vi "ADAM_scan_diagnostic.vi"() -> ()   [LabVIEW 2021]
uses:
  ADAM Client/Sub VIs/ADAM Controls/Ch_description_ADAM.ctl
  ADAM Client/Sub VIs/ADAM Controls/Module_type_ADAM.ctl
  ADAM Client/Sub VIs/ADAM Controls/Function_ADAM.ctl
  ADAM Client/Sub VIs/ADAM Controls/Channel_State.ctl
  ADAM Client/Sub VIs/ADAM Controls/Calib_type_ADAM.ctl
  ADAM Client/Sub VIs/ADAM Controls/Address.ctl
  ADAM_Global.vi
  Sub VI's/Channel_Description_Global.vi
panel:
  in  "deleteChannel":bool
  in  "reloadDescription":bool
  out "chTime(s)":dbl caption="Time taken" format="%_3ps"
  in  "Save Changes":bool
  in  "Simulate":enum32{"Scan Table", "Simulate"}(radio)
  in  "stop":bool
  in  "Value to Output":dbl format="%.2f"
  out "Value Read":dbl format="%.2f"
  out "Scan comment":string
  in  "Execute channel":bool
  in  "Select channel":bool
  in  "Ch Description":T1 {"Duty" format="%016b"; "D" format="%#_5g"; "C" format="%#_5g"; "B" format="%#_5g"; "A" format="%#_5g"}
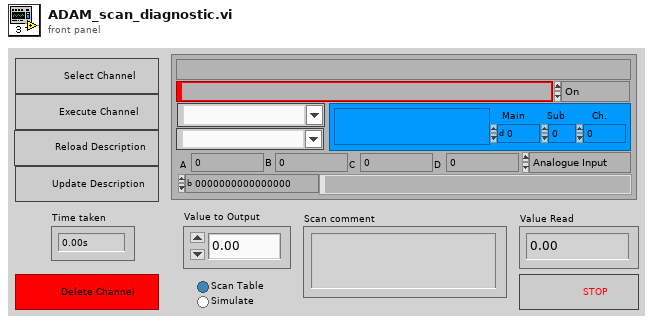
[diagram p1: front panel]
types:
  T1 = typedef "Ch_description_ADAM.ctl" = cluster{"Ch Name":string, "Type":T2, "Function":T3, "Ch State":T4, "Calibration type":T5, "A":dbl, "B":dbl, "C":dbl, "D":dbl, "Comments":string, "Address":T6, "String":string, "Duty":u16}
  T2 = typedef "Module_type_ADAM.ctl" = string
  T3 = typedef "Function_ADAM.ctl" = enum16{"Analogue Input", "Digital Input", "Event counter", "Event rate", "Analogue Output", "Digital Output", "Relay Output"}
  T4 = typedef "Channel_State.ctl" = enum16{"On", "Off", "Always On", "Always Off"}
  T5 = typedef "Calib_type_ADAM.ctl" = string
  T6 = typedef "Address.ctl" = cluster{"Main":i32, "Ch.":i32, "Sub":i32, "Port Name":string}
  T7 = enum16{"Load ADAM setup from excel file", "Save ADAM setup to excel file"}
  T8 = enum16{"Zero or one", "One", "Zero or more", "One or more"}
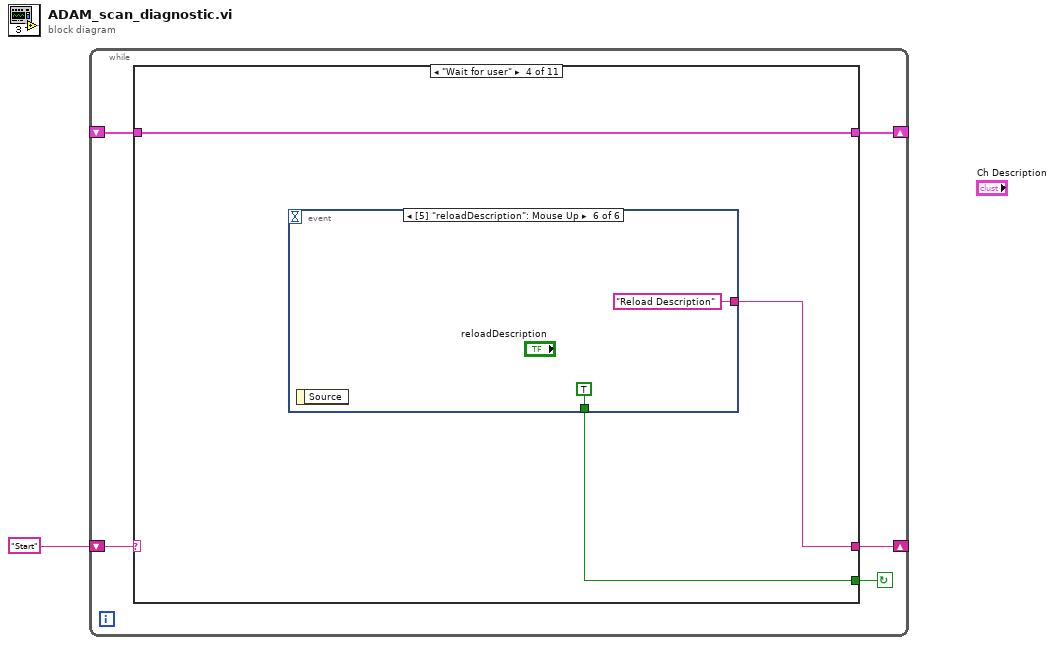
[diagram p0: block diagram]
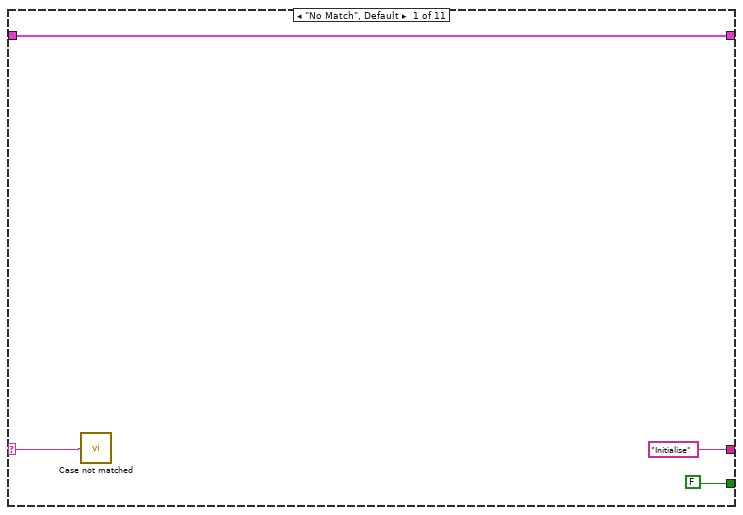
[diagram p2: hidden frame]
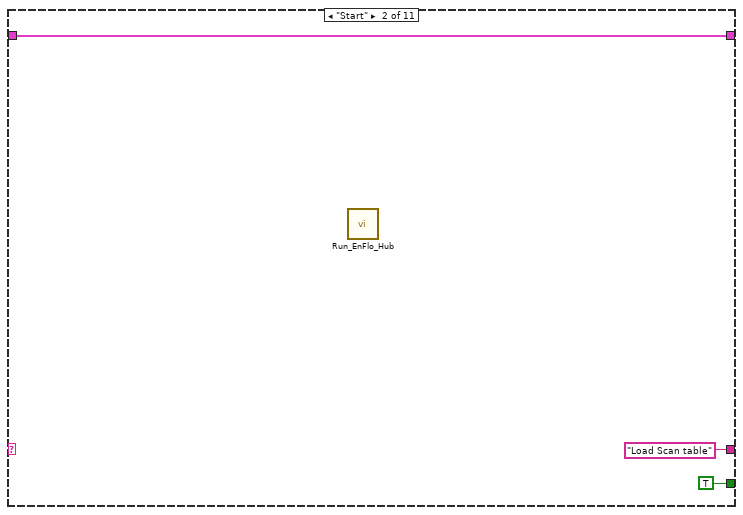
[diagram p3: hidden frame]
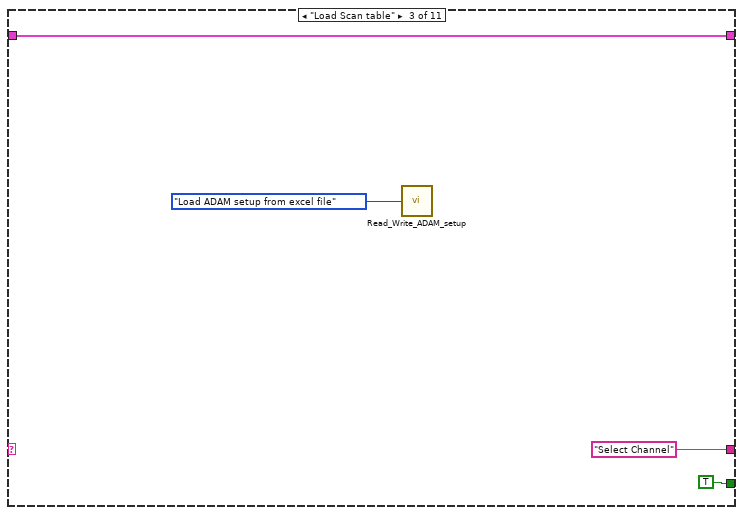
[diagram p4: hidden frame]
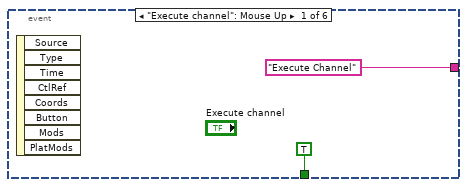
[diagram p5: hidden frame]
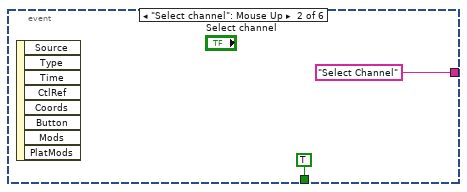
[diagram p6: hidden frame]
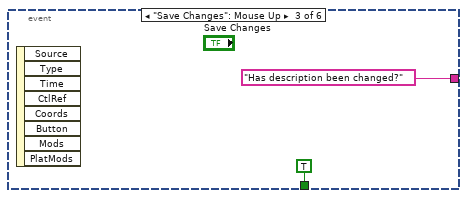
[diagram p7: hidden frame]
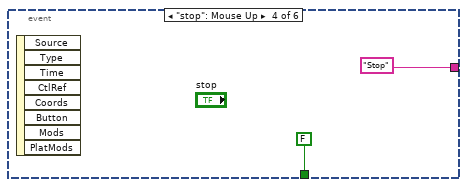
[diagram p8: hidden frame]
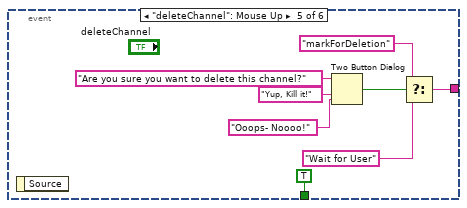
[diagram p9: hidden frame]
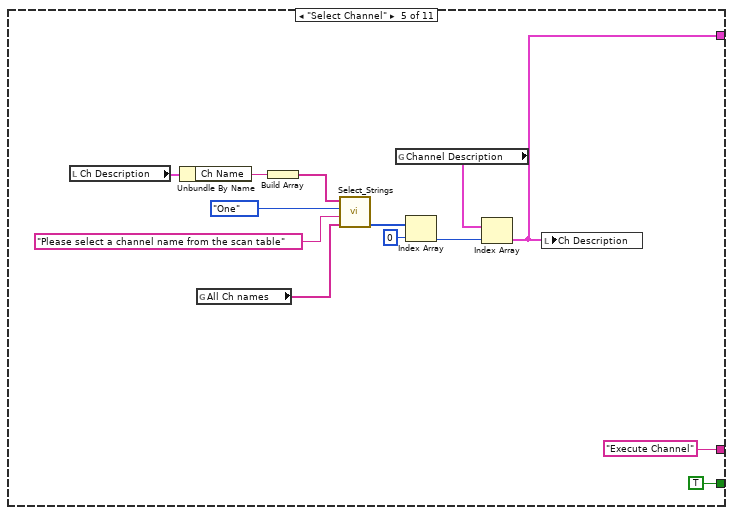
[diagram p10: hidden frame]
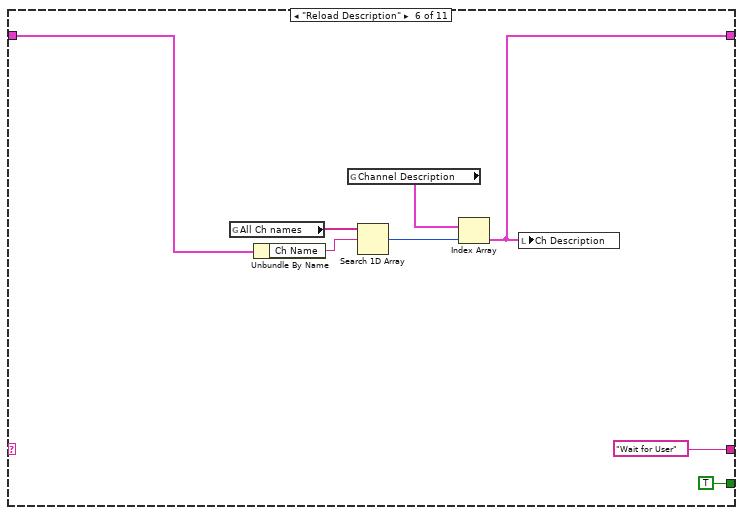
[diagram p11: hidden frame]
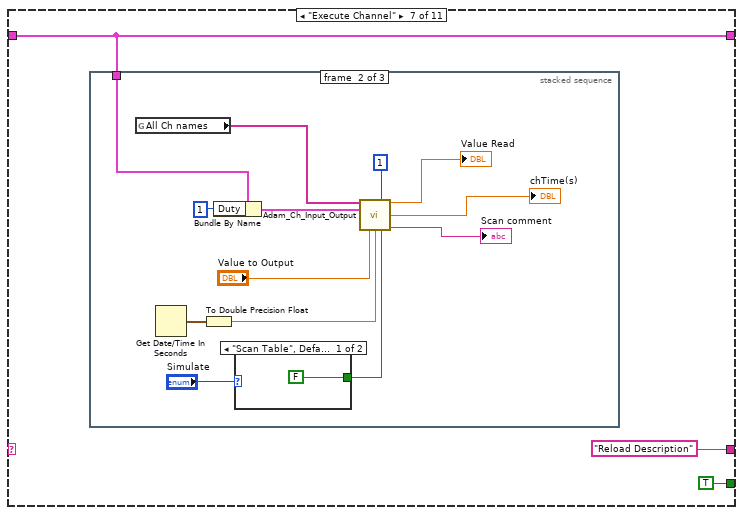
[diagram p12: hidden frame]
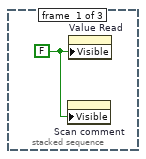
[diagram p13: hidden frame]
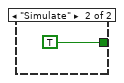
[diagram p14: hidden frame]
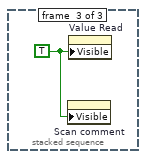
[diagram p15: hidden frame]
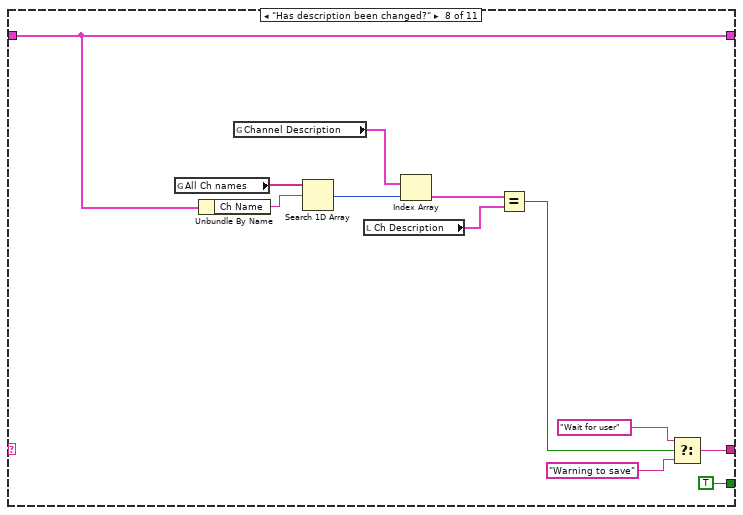
[diagram p16: hidden frame]
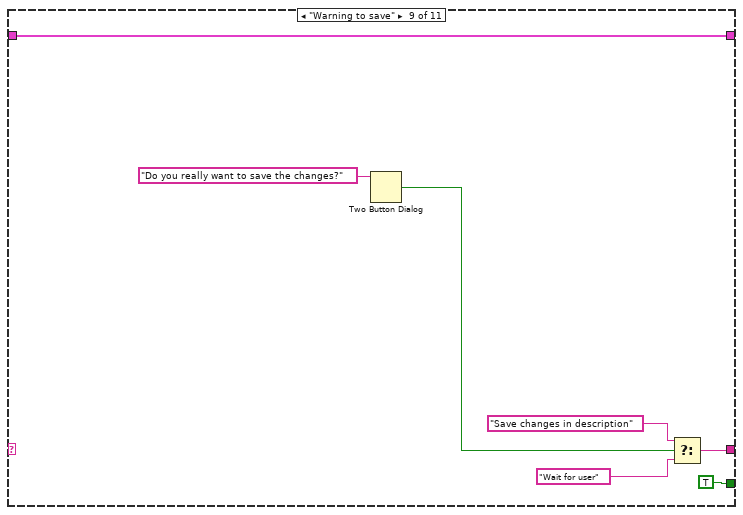
[diagram p17: hidden frame]
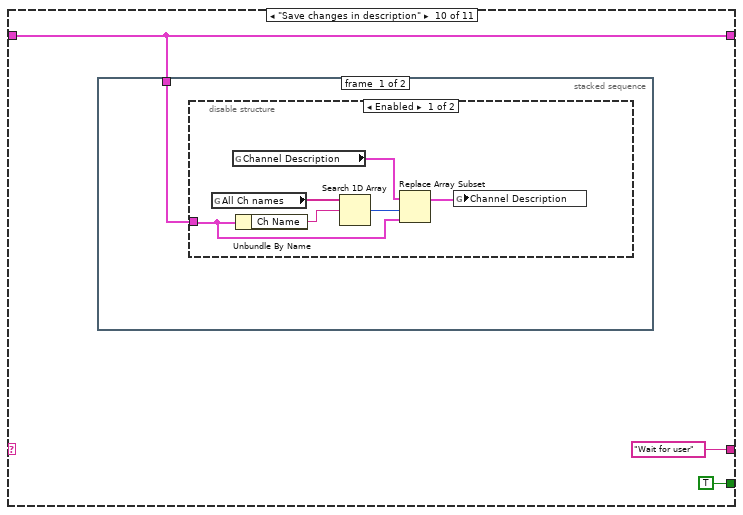
[diagram p18: hidden frame]
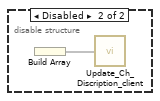
[diagram p19: hidden frame]
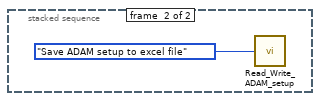
[diagram p20: hidden frame]
diagram:
  n1 = while {
    shift-left: "Start" -> [w4]
    shift-right: [w5] -> _
    shift-right: [w3] -> _
    shift-left: _ -> [w2]
    stop <- w6 continue-if-true
    n2 = case shown="\"Wait for user\"" w4 {
      selector: w4 -> [w8 _ _ _ _ _ _ _ _ _ _]
      tunnel: [FALSE TRUE TRUE w19 TRUE TRUE TRUE TRUE TRUE TRUE TRUE] -> w6
      tunnel: ["Initialise" "Load Scan table" "Select Channel" w20 "Execute Channel" "Wait for User" "Reload Description" w85 w97 "Wait for user" "Load Scan table"] -> w5
      tunnel: [w7 w11 w14 w18 w39 w52 w60 w81 w92 w99 w111] -> w3
      tunnel: w2 -> [w7 w11 w14 w18 _ w53 w60 w81 w92 w99 w111]
      frame "No Match", Default {
        n3 = call "Case not matched.vi"("Case Name not Matched"=w8) -> ()
      }
      frame "Start" {
        n4 = call "Run_EnFlo_Hub.vi"() -> ()  [unwired: 7 in, 1 out]
      }
      frame "Load Scan table" {
        n5 = call "Read_Write_ADAM_setup.vi"("Mode"=T7."Load ADAM setup from excel file") -> ()  [unwired: 4 in]
      }
      frame "Wait for user" {
        n6 = event shown="[5] \"reloadDescription\": Mouse Up" {
          selector: _ -> [_ _ _ _ _ _]
          dyn-events: _ -> [_ _ _ _ _ _]
          timeout: _ -> [_ _ _ _ _ _]
          tunnel: ["Execute Channel" "Select Channel" "Has description been changed?" "Stop" w33 "Reload Description"] -> w20
          tunnel: [TRUE TRUE TRUE FALSE TRUE TRUE] -> w19
          event "Execute channel": Mouse Up {
            n7 = event-data() -> ()  [unwired: 1 in, 8 out]
          }
          event "Select channel": Mouse Up {
            n8 = event-data() -> ()  [unwired: 1 in, 8 out]
          }
          event "Save Changes": Mouse Up {
            n9 = event-data() -> ()  [unwired: 1 in, 8 out]
          }
          event "stop": Mouse Up {
            n10 = event-data() -> ()  [unwired: 1 in, 8 out]
          }
          event "deleteChannel": Mouse Up {
            n11 = event-data() -> ()  [unwired: 1 in, 1 out]
            n12 = Two Button Dialog(message="Are you sure you want to delete this channel?", 1:"Ooops- Noooo!" ("F button name (\"Cancel\")"), 2:"Yup, Kill it!" ("T button name (\"OK\")")) -> (T button?=w32:bool)
            n13 = Select(t="markForDeletion", s=w32, f="Wait for User") -> (s? t:f=w33:string)
          }
          event "reloadDescription": Mouse Up {
            n14 = event-data() -> ()  [unwired: 1 in, 1 out]
          }
        }
      }
      frame "Select Channel" {
        n15 = local read "Ch Description"() -> (w43:T1)
        n16 = Unbundle By Name(w43) -> ("Ch Name"=w42:string)
        n17 = global read "ADAM_Global.vi" "All Ch names"() -> (w49:string[])
        n18 = Build Array(w42) -> (w41:string[])
        n19 = call "Select_Strings.vi"("Available Ch names"=w49, "Message"="Please select a channel name from the scan table", "Selector mode"=T8."One", "Desired Ch names (in)"=w41) -> ("Ch Indicies Chosen"=w45:i32[])  [unwired: 2 in, 2 out]
        n20 = global read "Channel_Description_Global.vi" "Channel Description"() -> (w44:T1[])
        n21 = Index Array(array=w45, index=0) -> (element=w40:i32)
        n22 = Index Array(array=w44, index=w40) -> (element=w39:T1)
        n23 = local write "Ch Description"(w39) -> ()
      }
      frame "Reload Description" {
        n24 = global read "ADAM_Global.vi" "All Ch names"() -> (w56:string[])
        n25 = Unbundle By Name(w53) -> ("Ch Name"=w55:string)
        n26 = global read "Channel_Description_Global.vi" "Channel Description"() -> (w57:T1[])
        n27 = Search 1D Array(1D array=w56, element=w55) -> (index of element=w54:i32)  [unwired: 1 in]
        n28 = Index Array(array=w57, index=w54) -> (element=w52:T1)
        n29 = local write "Ch Description"(w52) -> ()
      }
      frame "Execute Channel" {
        n30 = stacked-sequence {
          tunnel: w60 -> [_ w64 _]
          frame #0 {
            w63 = FALSE ("Visible")
            n31 = property on="Scan comment" class="Str"("Visible"=w63) -> ()  [unwired: 2 in, 2 out]
            n32 = property on="Value Read" class="DigNum (strict)"("Visible"=w63) -> ()  [unwired: 2 in, 2 out]
          }
          frame #1 {
            n33 = global read "ADAM_Global.vi" "All Ch names"() -> (w71:string[])
            n34 = Get Date/Time In Seconds() -> (seconds since 1Jan1904=w69:timestamp)
            n35 = To Double Precision Float(number=w69) -> (double precision float=w68:dbl)
            n36 = Bundle By Name(cluster=w64, "Duty"=u16 1 ("Duty No")) -> (w72:T1)
            n37 = case shown="\"Scan Table\", Default" "Simulate" {
              tunnel: [FALSE TRUE] -> w65
              frame "Scan Table", Default {
              }
              frame "Simulate" {
              }
            }
            n38 = call "Adam_Ch_Input_Output.vi"("Ch names"=w71, "Duty No"=u16 1, "Ch Description"=w72, "Value to Output"="Value to Output", "Current Time (sec)"=w68, "Simulate"=w65) -> ("Calibrated units"=→"Value Read":dbl, "chTime(s)"=→"chTime(s)":dbl, "Scan comment"=→"Scan comment":string)  [unwired: 5 in, 2 out]
          }
          frame #2 {
            w79 = TRUE ("Visible")
            n39 = property on="Scan comment" class="Str"("Visible"=w79) -> ()  [unwired: 2 in, 2 out]
            n40 = property on="Value Read" class="DigNum (strict)"("Visible"=w79) -> ()  [unwired: 2 in, 2 out]
          }
        }
      }
      frame "Has description been changed?" {
        n41 = global read "ADAM_Global.vi" "All Ch names"() -> (w83:string[])
        n42 = Unbundle By Name(w81) -> ("Ch Name"=w82:string)
        n43 = global read "Channel_Description_Global.vi" "Channel Description"() -> (w90:T1[])
        n44 = Search 1D Array(1D array=w83, element=w82) -> (index of element=w80:i32)  [unwired: 1 in]
        n45 = local read "Ch Description"() -> (w88:T1)
        n46 = Index Array(array=w90, index=w80) -> (element=w89:T1)
        n47 = Equal?(x=w89, y=w88) -> (x = y?=w87:bool)
        n48 = Select(t="Wait for user", s=w87, f="Warning to save") -> (s? t:f=w85:string)
      }
      frame "Warning to save" {
        n49 = Two Button Dialog(message="Do you really want to save the changes?") -> (T button?=w95:bool)  [unwired: 2 in]
        n50 = Select(t="Save changes in description" ("f"), s=w95, f="Wait for user") -> (s? t:f=w97:string)
      }
      frame "Save changes in description" {
        n51 = stacked-sequence {
          tunnel: w99 -> [w102 _]
          frame #0 {
            n52 = disable-structure shown="Enabled" {
              disable-tunnel: w102 -> [w104 _]
              frame Enabled {
                n53 = global read "ADAM_Global.vi" "All Ch names"() -> (w106:string[])
                n54 = global read "Channel_Description_Global.vi" "Channel Description"() -> (w108:T1[])
                n55 = Unbundle By Name(w104) -> ("Ch Name"=w105:string)
                n56 = Search 1D Array(1D array=w106, element=w105) -> (index of element=w103:i32)  [unwired: 1 in]
                n57 = Replace Array Subset(array=w108, new element=w104, index=w103) -> (w107:T1[])
                n58 = global write "Channel_Description_Global.vi" "Channel Description"(w107) -> ()
              }
              frame Disabled {
                n59 = Build Array() -> (w109:void[])  [unwired: 1 in]
                n60 = call "Update_Ch_Discription_client.vi"("Channels to update In"=w109) -> ()  [unwired: 1 in]
              }
            }
          }
          frame #1 {
            n61 = call "Read_Write_ADAM_setup.vi"("Mode"=T7."Save ADAM setup to excel file") -> ()  [unwired: 4 in]
          }
        }
      }
      frame "markForDeletion" {
        n62 = stacked-sequence {
          tunnel: w111 -> [w114 _]
          frame #0 {
            n63 = disable-structure shown="Enabled" {
              disable-tunnel: w114 -> [w115 _]
              frame Enabled {
                n64 = global read "ADAM_Global.vi" "All Ch names"() -> (w120:string[])
                n65 = Unbundle By Name(w115) -> ("Ch Name"=w119:string)
                n66 = global read "Channel_Description_Global.vi" "Channel Description"() -> (w122:T1[])
                n67 = Bundle By Name(cluster=w115, "Address.Port Name"="DELETE") -> (w116:T1)
                n68 = Search 1D Array(1D array=w120, element=w119) -> (index of element=w118:i32)  [unwired: 1 in]
                n69 = Replace Array Subset(array=w122, new element=w116, index=w118) -> (w121:T1[])
                n70 = global write "Channel_Description_Global.vi" "Channel Description"(w121) -> ()
              }
              frame Disabled {
                n71 = Build Array() -> (w123:void[])  [unwired: 1 in]
                n72 = call "Update_Ch_Discription_client.vi"("Channels to update In"=w123) -> ()  [unwired: 1 in]
              }
            }
          }
          frame #1 {
            n73 = local write "Ch Description"(T1 {"Ch Name"="", "Type"="", "Function"=enum."Analogue Input", "Ch State"=enum."On", "Calibration type"="", "A"=0.0, "B"=0.0, "C"=0.0, "D"=0.0, "Comments"="", "Address"={"Main"=0, "Ch."=0, "Sub"=0, "Port Name"=""}, "String"="", "Duty"=0} ("Ch Description")) -> ()
            n74 = call "Read_Write_ADAM_setup.vi"("Mode"=T7."Save ADAM setup to excel file") -> ()  [unwired: 4 in]
          }
        }
      }
    }
  }
